vi "PhaseDelta.vi"(10 "Plot 1":u16[](array[numeric]), 11 "Plot 0":u16[](array[numeric])) -> (3 "Phase Delta":dbl)   [LabVIEW 2017]
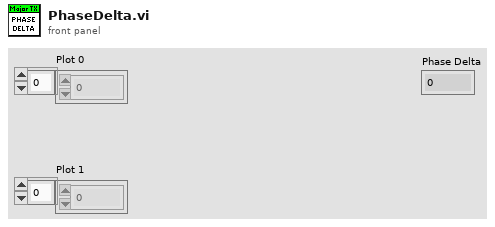
[diagram p1: front panel]
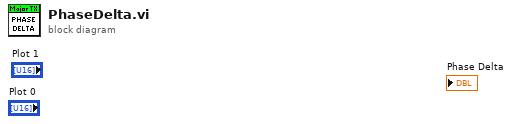
[diagram p0: block diagram]
diagram:
